vi "dataset.add.vi"(6 "Series Tags":map{string, string}(c390), 8 "error in":errorcluster, 9 "refName":string, 10 "Dataset RID":string, 11 "asset in":refnum<class "asset.lvclass">) -> (0 "error out":errorcluster, 3 "asset out":refnum<class "asset.lvclass">)   [LabVIEW 2020, in "asset.lvclass"]
uses:
  asset.lvclass
  Nominal Client/Nominal Client.lvclass
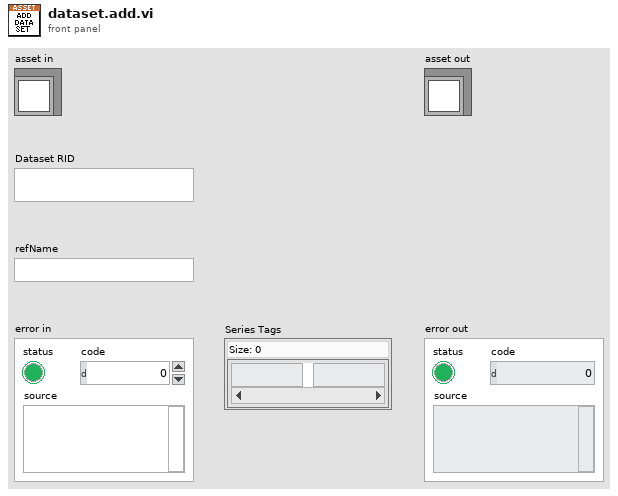
[diagram p1: front panel]
types:
  T1 = typedef "dataScopes.lvlib/links.ctl" = cluster{"URL":string, "Title":string}[]
  T2 = typedef "dataScopes.lvlib/data_scopes.ctl" = T3[]
  T3 = typedef "dataScopes.lvlib/data_scope.ctl" = cluster{"dataScopeName":string, "dataSource":T4, "seriesTags":map{string, string}, "offset":T6}
  T4 = typedef "dataScopes.lvlib/data_source.ctl" = cluster{"type":T5, "rid":string}
  T5 = typedef "dataScopes.lvlib/type.ctl" = enum16{"dataset", "connection", "logSet", "video"}
  T6 = typedef "dataScopes.lvlib/offset.ctl" = cluster{"seconds":i32, "nanos":i32, "picos":i32}
  T7 = cluster{"rid":string, "title":string, "properties":refnum<class "properties.lvclass">, "labels":refnum<class "labels.lvclass">, "Links":T1, "datascopes":T2, "createdAt":timestamp, "updatedAt":timestamp, "attachments":refnum<class "labels.lvclass">, "isStaged":bool, "isArchived":bool, "description":string, "createdBy":string, "type":string}
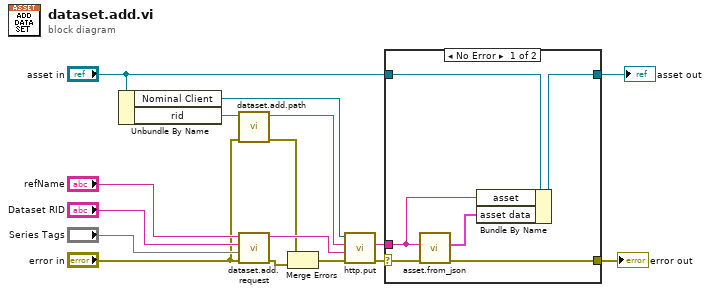
[diagram p0: block diagram]
diagram:
  n1 = Unbundle By Name("asset in") -> ("Nominal Client"=w16:refnum<class "Nominal Client.lvclass">, "rid"=w6:string)
  n2 = call "dataset.add.path.vi"("error in"="error in", "Asset RID"=w6) -> ("error out"=w3:errorcluster, "Path"=w5:string)  [unwired: 8 in]
  n3 = call "dataset.add.request.vi"("error in"="error in", "Series Tags"="Series Tags", "Dataset RID"="Dataset RID", "refName"="refName") -> ("error out"=w2:errorcluster, "Request"=w7:string)  [unwired: 6 in]
  n4 = Merge Errors(w3, w2) -> (w1:errorcluster)
  n5 = call "http.put.vi"("error in"=w1, "Body"=w7, "Path"=w5, "Nominal Client in"=w16) -> ("error out"=w15:errorcluster, "Response"=w12:string)  [unwired: 4 in, 2 out]
  n6 = case shown="No Error" w15 {
    selector: w15 -> [w22 w24]
    tunnel: [w21 w24] -> w14
    tunnel: "asset in" -> [w20 w23]
    tunnel: w12 -> [w18 _]
    tunnel: [w17 w23] -> w11
    frame No Error {
      n7 = call "asset.from_json.vi"("error in"=w22, "asset"=w18) -> ("error out"=w21:errorcluster, "Asset Data"=w19:T7)  [unwired: 8 in]
      n8 = Bundle By Name(cluster=w20, "asset"=w18, "asset data"=w19) -> (w17:refnum<class "asset.lvclass">)
    }
    frame Error {
    }
  }
  "asset out" <- w11
  "error out" <- w14
